vi "Init.vi"(8 "error in":errorcluster, 10 "Sourcegrid Container":refnum<k24>(container), 11 "Grid in":refnum<class "SourceGrid.lvclass">) -> (0 "error out":errorcluster, 3 "Grid out":refnum<class "SourceGrid.lvclass">)   [LabVIEW 2024, in "SourceGrid.lvlib" / "SourceGrid.lvclass"]
uses:
  SourceGrid.lvclass
  SourceGrid.lvclass/SourceGrid.ctl
  D:/git/Sourcegrid-LabVIEW/dll/SourceGrid.dll
  dll/SourceGrid.dll
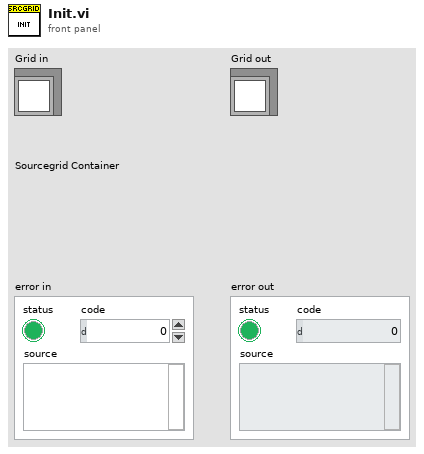
[diagram p1: front panel]
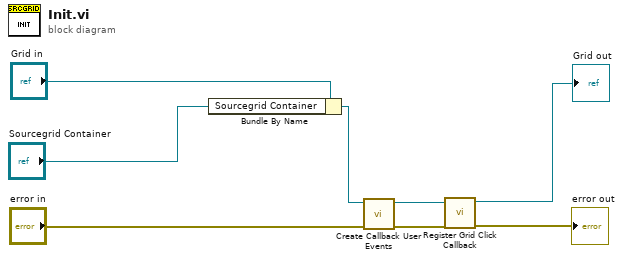
[diagram p0: block diagram]
diagram:
  n1 = Bundle By Name(cluster="Grid in", "Sourcegrid Container"="Sourcegrid Container") -> (w5:refnum<class "SourceGrid.lvclass">)
  n2 = call-dynamic "Create Callback User Events.vi"("error in"="error in", "SourceGrid in"=w5) -> ("error out"=w3:errorcluster, "SourceGrid out"=w4:refnum<class "SourceGrid.lvclass">)  [unwired: 8 in]
  n3 = call-dynamic "Register Grid Click Callback.vi"("error in"=w3, "SourceGrid in"=w4) -> ("error out"=→"error out":errorcluster, "SourceGrid out"=→"Grid out":refnum<class "SourceGrid.lvclass">)  [unwired: 8 in]
